vi "Parse.vi"(8 "Error In":errorcluster, 11 "object in":refnum<class "2021_13.lvclass">) -> (0 "Error Out":errorcluster, 3 "object out":refnum<class "2021_13.lvclass">)   [LabVIEW 2020, in "2021_13.lvclass"]
uses:
  2021_13.lvclass
  2021_13.lvclass/2021_13.ctl
panel:
  out "Array 2":cluster{"Fold":enum16{"X", "Y"}, i32}[](array[cluster])
  out "Array":bool[][](array[boolean])
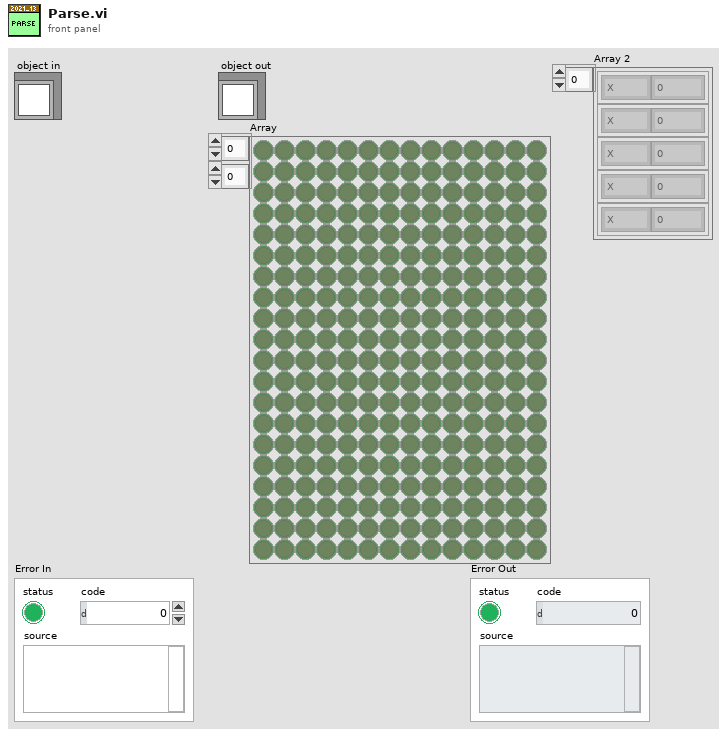
[diagram p1: front panel]
diagram:
  (unwired) "6,10\n0,14\n9,10\n0,3\n10,4\n4,11\n6,0\n6,12\n4,1\n0,13\n10,12\n3,4\n3,0\n8,4\n1,10\n2,14\n8,10\n9,0\n\nfold along y=7\nfold along x=5" ("regular expression")
  n1 = Match Pattern(string="176,226\n749,474\n1218,784\n1193,451\n478,224\n1019,620\n865,667\n884,178\n622,505\n43,856\n475,619\n1295,96\n497,499\n589,326\n117,267\n559,361\n402,863\n1220,277\n167,617\n955,560\n1011,135\n311,618\n865,198\n855,761\n698,241\n180,786\n728,523\n832,222\n865,67\n1280,649\n155,844\n990,406\n688,505\n990,488\n1116,288\n1047,266\n181,408\n27,401\n883,257\n253,610\n1213,131\n967,395\n581,605\n316,302\n1260,425\n967,171\n721,774\n618,668\n604,51\n858,323\n520,553\n271,730\n749,567\n1274,892\n1054,102\n117,301\n201,598\n227,257\n1193,267\n146,658\n87,498\n1017,313\n1211,628\n118,668\n1059,259\n48,169\n698,292\n405,516\n676,110\n1101,667\n298,453\n251,119\n1046,529\n1245,774\n1019,722\n1009,365\n117,593\n27,469\n599,164\n915,775\n1088,91\n530,407\n124,571\n494,378\n97,59\n995,443\n311,49\n345,822\n175,469\n174,560\n427,66\n261,120\n371,38\n73,844\n145,637\n674,675\n1275,646\n787,44\n1074,57\n478,229\n1140,630\n999,51\n559,252\n30,649\n1256,182\n836,882\n801,679\n271,394\n176,665\n989,211\n887,533\n431,147\n760,539\n1207,523\n73,172\n786,690\n504,674\n1039,858\n1034,702\n540,277\n457,89\n393,436\n995,397\n728,371\n556,850\n180,747\n345,72\n887,361\n484,742\n692,598\n835,619\n1057,158\n1159,891\n412,201\n801,33\n391,628\n1116,736\n1240,344\n530,487\n667,397\n639,171\n880,168\n390,813\n788,176\n1250,793\n780,487\n445,667\n1217,857\n832,705\n42,763\n813,499\n700,444\n114,619\n1191,884\n119,10\n791,313\n917,436\n1243,343\n1290,513\n15,798\n728,75\n179,833\n683,873\n773,260\n830,271\n567,620\n610,450\n395,567\n231,361\n1135,469\n1278,46\n1136,399\n780,357\n403,567\n671,778\n343,51\n902,78\n676,241\n345,486\n504,224\n136,593\n458,400\n806,224\n274,873\n753,347\n591,714\n699,856\n966,427\n991,773\n169,859\n85,339\n817,175\n470,733\n932,52\n378,310\n164,694\n999,619\n552,168\n523,44\n807,303\n843,623\n999,299\n160,826\n97,723\n557,347\n790,553\n1143,617\n701,637\n1109,598\n1193,515\n418,505\n522,649\n184,733\n801,705\n227,42\n1255,235\n222,159\n92,784\n95,364\n912,344\n85,787\n1170,511\n756,809\n473,184\n226,731\n676,513\n1130,108\n251,775\n219,484\n219,708\n151,357\n1192,674\n360,505\n1267,486\n972,592\n626,221\n1268,292\n445,248\n830,495\n69,143\n401,485\n1213,884\n1175,313\n1241,303\n612,627\n634,676\n947,620\n729,498\n721,326\n1299,451\n544,537\n1079,306\n373,172\n1036,873\n519,357\n1163,203\n1197,268\n802,147\n95,585\n181,413\n858,213\n604,537\n452,323\n662,488\n276,401\n1178,357\n743,128\n236,57\n1210,309\n905,516\n99,492\n430,168\n1083,637\n706,625\n345,408\n569,555\n831,61\n32,400\n1208,352\n892,505\n97,884\n58,7\n227,852\n1143,572\n643,751\n311,548\n12,450\n276,394\n505,707\n370,355\n599,659\n445,67\n557,884\n1211,154\n1084,137\n1238,523\n551,747\n264,589\n755,850\n887,431\n311,845\n27,465\n254,814\n102,726\n10,750\n184,676\n676,784\n831,541\n1039,500\n937,172\n140,607\n831,353\n479,61\n264,813\n259,119\n840,733\n239,262\n1136,750\n68,341\n1275,248\n445,26\n766,537\n1265,396\n1098,53\n774,668\n50,537\n152,175\n118,674\n472,331\n1283,401\n1299,443\n1163,691\n1012,493\n909,50\n639,723\n870,393\n975,185\n1212,492\n229,777\n1310,172\n627,149\n42,292\n1206,287\n136,145\n97,131\n11,443\n671,171\n335,325\n686,549\n44,444\n1059,119\n1208,726\n197,420\n1120,301\n753,803\n1215,642\n975,709\n564,281\n197,474\n207,150\n805,707\n552,253\n144,563\n556,716\n1083,497\n503,357\n271,500\n1268,602\n145,215\n756,163\n290,296\n589,120\n1176,341\n691,198\n535,296\n962,625\n296,574\n555,873\n445,446\n171,722\n932,584\n944,401\n955,807\n580,479\n723,103\n355,334\n910,814\n73,624\n971,3\n698,653\n202,547\n1295,723\n1083,66\n283,436\n65,777\n295,738\n751,361\n1190,750\n519,177\n991,26\n494,826\n95,82\n1084,731\n1083,257\n1027,436\n1213,579\n75,150\n792,77\n518,77\n704,171\n72,523\n1116,158\n306,513\n388,65\n315,443\n97,619\n93,663\n282,892\n112,254\n134,647\n373,274\n113,268\n69,420\n151,751\n426,626\n1178,494\n473,486\n1211,413\n1119,465\n519,313\n691,795\n535,598\n170,712\n831,93\n1299,133\n1266,444\n937,786\n125,184\n718,813\n423,431\n229,290\n440,393\n1074,281\n1197,178\n965,72\n214,501\n263,621\n922,9\n788,649\n306,558\n909,284\n55,730\n1207,371\n1198,469\n994,302\n263,721\n311,299\n104,287\n550,355\n391,714\n216,331\n808,175\n1265,498\n694,855\n749,409\n746,613\n212,53\n378,584\n1026,355\n145,355\n425,604\n132,357\n557,507\n1047,621\n1159,3\n284,66\n1026,592\n28,553\n257,143\n470,228\n309,408\n315,497\n530,805\n882,611\n1113,420\n372,892\n1165,705\n892,11\n1236,479\n683,745\n20,513\n447,150\n753,507\n1290,558\n251,635\n721,120\n1193,739\n60,218\n309,486\n927,858\n509,705\n1178,537\n320,488\n1032,501\n618,598\n1034,500\n344,19\n763,858\n892,883\n1292,667\n561,679\n99,266\n774,226\n113,324\n627,877\n671,723\n907,567\n1056,841\n100,507\n253,64\n1237,605\n38,407\n1034,425\n654,172\n445,491\n348,625\n1233,128\n832,224\n445,448\n401,284\n140,511\n554,809\n1088,735\n567,498\n1116,437\n1135,751\n730,479\n581,50\n967,51\n709,745\n370,715\n32,46\n231,306\n209,739\n67,343\n837,315\n1196,723\n98,402\n1036,425\n98,850\n1233,340\n946,2\n1292,227\n1225,339\n920,529\n1283,465\n284,539\n1079,809\n868,53\n1059,567\n780,537\n171,172\n1215,812\n468,287\n1059,635\n401,50\n479,833\n999,49\n587,791\n611,486\n977,824\n343,52\n1303,284\n1017,784\n574,526\n1165,215\n127,722\n253,158\n512,228\n612,205\n643,397\n927,659\n1300,144\n1126,676\n1299,751\n80,424\n1200,537\n692,296\n535,436\n641,855\n919,714\n223,299\n725,591\n1213,723\n658,516\n838,331\n826,294\n1267,856\n470,653\n97,212\n837,710\n756,835\n831,425\n502,175\n290,2\n319,773\n1049,355\n919,833\n591,845\n373,786\n636,219\n540,802\n1257,597\n478,222\n298,1\n28,341\n850,9\n184,666\n251,327\n554,835\n995,891\n848,190\n1087,147\n1282,553\n152,560\n1236,415\n879,147\n674,219\n591,180\n370,144\n293,110\n1159,751\n940,592\n1073,830\n97,275\n503,21\n321,742\n1176,647\n1243,418\n107,858\n840,666\n281,219\n1265,189\n97,579\n291,620\n67,418\n749,679\n278,501\n272,182\n319,26\n1193,634\n6,488\n1001,408\n1131,61\n20,336\n666,750\n223,147\n1255,164\n1197,324\n20,241\n1139,722\n940,403\n627,45\n366,407\n363,172\n126,668\n1004,336\n711,164\n534,144\n773,525\n610,444\n520,647\n6,600\n455,133\n759,747\n766,357\n509,355\n759,147\n692,2\n1268,355\n530,313\n325,119\n117,379\n711,730\n753,91\n760,735\n1211,292\n775,296\n420,782\n338,592\n706,537\n465,697\n460,9\n503,143\n428,78\n1193,155\n1220,617\n1217,791\n528,226\n355,87\n1044,885\n801,579\n536,226\n145,539\n388,9\n551,147\n1155,844\n1012,45\n1260,619\n431,523\n1034,873\n84,873\n74,479\n691,696\n202,213\n229,499\n353,529\n643,451\n194,288\n169,35\n38,39\n93,499\n54,182\n966,19\n790,229\n170,630\n132,89\n1215,687\n1260,537\n1038,40\n175,21\n55,164\n425,731\n1101,739\n753,884\n793,107\n321,11\n922,829\n1081,499\n1079,85\n883,66\n194,736\n547,858\n356,893\n465,197\n540,275\n791,357\n522,89\n865,827\n38,597\n59,75\n135,313\n50,843\n749,215\n311,346\n378,52\n325,775\n775,744\n669,855\n683,149\n487,870\n1245,120\n1081,395\n769,122\n1282,445\n190,301\n1178,649\n946,892\n42,539\n1283,493\n209,369\n1196,171\n753,547\n529,184\n1146,200\n823,277\n647,284\n567,128\n107,36\n517,787\n423,361\n644,750\n1252,7\n333,294\n1217,26\n1303,610\n45,396\n175,61\n920,813\n952,544\n522,718\n848,359\n348,241\n1046,589\n263,861\n791,537\n356,1\n868,617\n1049,774\n823,572\n301,365\n634,381\n442,841\n1198,254\n27,493\n1283,849\n432,735\n33,558\n875,708\n38,855\n770,725\n263,609\n361,110\n1272,39\n729,172\n363,620\n1083,738\n908,31\n910,53\n848,862\n1178,89\n1010,369\n509,691\n72,11\n69,474\n676,676\n281,257\n1113,474\n544,357\n1174,593\n348,65\n38,465\n1260,394\n760,159\n145,189\n731,744\n266,885\n971,397\n181,481\n634,218\n103,523\n816,378\n1242,789\n145,257\n999,276\n1186,123\n\nfold along x=655\nfold along y=447\nfold along x=327\nfold along y=223\nfold along x=163\nfold along y=111\nfold along x=81\nfold along y=55\nfold along x=40\nfold along y=27\nfold along y=13\nfold along y=6" ("PuzzleInput"), regular expression="[\\r\\n][\\r\\n]") -> (before substring=w18:string, after substring=w17:string)  [unwired: 1 in, 2 out]
  n2 = call <userlib>:"Multi-line String to Array__ogtk.vi"("string"=w17) -> ("lines"=w16:string[])
  n3 = Spreadsheet String To Array(delimiter (Tab)=",", format string="%d", spreadsheet string=w18, array type (2D Dbl)=i32[][] []) -> (array=w11:i32[][])
  n4 = Index Array(array=w11, index (col) #1=0 ("disabled index (col)")) -> (element #1=w9:i32[], element #2=w7:i32[])  [unwired: 3 in]
  n5 = To Upper Case(1:w16) -> (0:w6:string[])
  n6 = for {
    tunnel: w6 -> [w31] mode=indexing
    tunnel: [w26] -> w4 mode=indexing
    (unwired) 0 ("Index")
    n7 = Scan From String(format string="FOLD ALONG %1s=%d", input string=w31, default 1=enum16{"X", "Y"}."X" ("Fold")) -> (output 1=w28:enum16{"X", "Y"}, output 2=w27:i32)  [unwired: 3 in, 3 out]
    n8 = Bundle("Fold"=w28, w27) -> (w26:cluster{"Fold":enum16{"X", "Y"}, i32})  [unwired: 1 in]
  }
  "Array 2" <- w4
  n9 = Array Max & Min(array=w9) -> (max value=w15:i32)  [unwired: 3 out]
  n10 = Array Max & Min(array=w7) -> (max value=w8:i32)  [unwired: 3 out]
  n11 = Increment(x=w15) -> (x+1=w14:i32)
  n12 = Increment(x=w8) -> (x+1=w2:i32)
  n13 = Increment(x=w2) -> (x+1=w1:i32)
  n14 = Initialize Array(FALSE, w1, w14) -> (w12:bool[][])
  n15 = for {
    tunnel: w11 -> [w35] mode=indexing
    shift-right: [w36] -> w5
    shift-left: w12 -> [w37]
    n16 = Index Array(array=w35) -> (element #1=w34:i32, element #2=w33:i32)  [unwired: 2 in]
    n17 = Replace Array Subset(array=w37, new element=TRUE ("new element/subarray"), index (row)=w33, index (col)=w34) -> (w36:bool[][])
  }
  "Array" <- w5
  n18 = Bundle By Name(cluster="object in", "Map"=w5, "Fold"=w4) -> (→"object out":refnum<class "2021_13.lvclass">)
  "Error Out" <- "Error In"
